vi "set specification file.vi"(8 "error in (no error)":errorcluster, 11 "spec_file":string) -> (0 "error out":errorcluster)   [LabVIEW 2019, in "libSimulationControl.lvlib"]
doc: "void set_specification_file(const char* spec_file);"
uses:
  libSimulationControl.lvlib
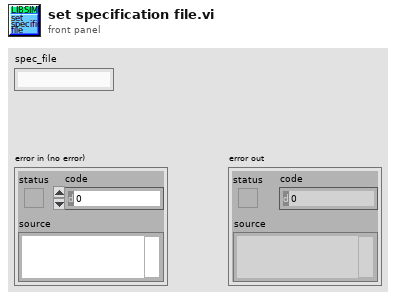
[diagram p1: front panel]
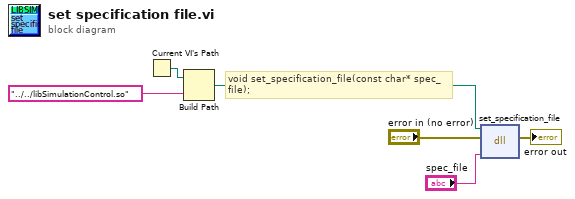
[diagram p0: block diagram]
diagram:
  # "void set_specification_file(const char* spec_file);"
  n1 = Current VI's Path() -> (path=w3:path)
  n2 = Build Path(base path=w3, name or relative path="../../libSimulationControl.so") -> (appended path=w1:path)
  n3 = dll-call lib="home/paul/Schreibtisch/Biogas_plant_setup/LabView/lib/libSimulationControl/libSimulationControl.*" fn="set_specification_file"(path in=w1, error in="error in (no error)", "spec_file"="spec_file") -> (error out=→"error out":errorcluster)  [unwired: 3 in, 1 out]
